vi "Store Error Queue.vi"(8 "error in (no error)":errorcluster, 11 "Error Handler Queue":refnum<class "Message Enqueuer.lvclass">) -> (0 "error out":errorcluster)   [LabVIEW 2015, in "Mag Lab Error Handler.lvlib" / "Mag Lab Error Handler.lvclass"]
uses:
  Mag Lab Error Handler.lvclass
  <vilib>/ActorFramework/Message Enqueuer/Message Enqueuer.lvclass
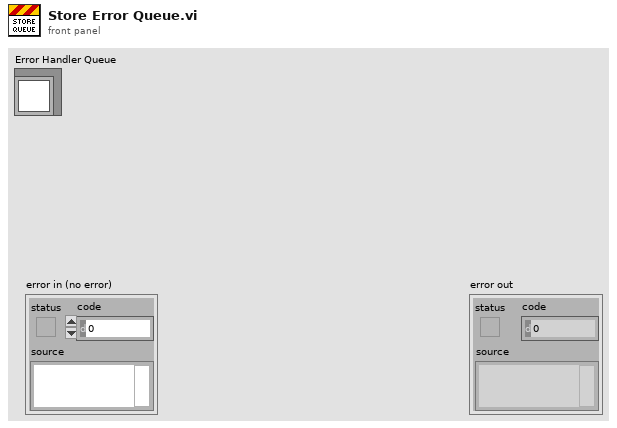
[diagram p1: front panel]
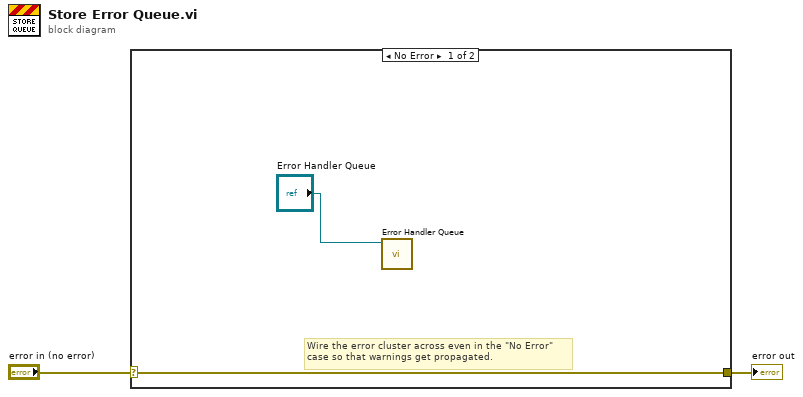
[diagram p0: block diagram]
diagram:
  n1 = case shown="No Error" "error in (no error)" {
    selector: "error in (no error)" -> [w4 w5]
    tunnel: [w4 w5] -> w1
    frame No Error {
      # "Wire the error cluster across even in the \"No Error\"\ncase so that warnings get propagated."
      n2 = call "Error Handler Queue.vi"("Error Handler Queue"="Error Handler Queue") -> ()  [unwired: 10 in, 1 out]
    }
    frame Error {
    }
  }
  "error out" <- w1
